vi "Configure TRIP.vi"(7 "All Channels (F)":bool, 8 "error in (no error)":errorcluster, 9 "Trip (0.00 s)":sgl format="%.2g", 10 "Channel (0)":u8, 11 "BoardHandle":T1) -> (0 "error out":errorcluster, 3 "BoardHandle out":T1)   [LabVIEW 2019, in "CAEN PSM.lvlib"]
doc: "This function allows to configure Ouput Trip time."
uses:
  CAEN PSM.lvlib
  Private/BoardHandle.ctl
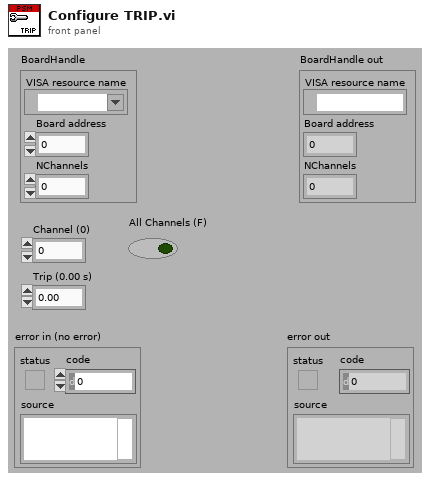
[diagram p1: front panel]
types:
  T1 = typedef "CAEN PSM.lvlib/BoardHandle.ctl" = cluster{"VISA resource name":refnum<visa-resource-name>, "Board address":u8, "NChannels":u8}
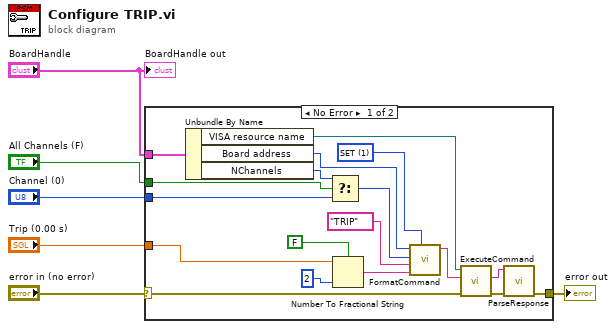
[diagram p0: block diagram]
diagram:
  n1 = case shown="No Error" "error in (no error)" {
    selector: "error in (no error)" -> [w12 w25]
    tunnel: "All Channels (F)" -> [w22 _]
    tunnel: "Channel (0)" -> [w20 _]
    tunnel: [w15 w25] -> w3
    tunnel: "BoardHandle" -> [w13 _]
    tunnel: "Trip (0.00 s)" -> [w7 _]
    frame No Error {
      w23 = u8 1 items=["MON", "SET"] ("CMD")
      n2 = Unbundle By Name(w13) -> ("VISA resource name"=w18:refnum<visa-resource-name>, "Board address"=w24:u8, "NChannels"=w21:u8)
      n3 = Select(t=w21, s=w22, f=w20) -> (s? t:f=w19:u8)
      n4 = Number To Fractional String(use system decimal point (T)=FALSE, number=w7, precision (6)=i16 2) -> (F-format string=w8:string)  [unwired: 1 in]
      n5 = call "FormatCommand.vi"("CMD (MON)"=w23, "VAL"=w8, "PAR"="TRIP", "CH"=w19, "BD (0)"=w24) -> ("cmd"=w17:string)  [unwired: 6 in]
      n6 = call "ExecuteCommand.vi"("error in (no error)"=w12, "Command"=w17, "VISA resource name"=w18) -> ("error out"=w16:errorcluster, "Response"=w14:string)  [unwired: 6 in, 1 out]
      n7 = call "ParseResponse.vi"("error in (no error)"=w16, "Response"=w14) -> ("error out"=w15:errorcluster)  [unwired: 6 in, 3 out]
    }
    frame Error {
    }
  }
  "error out" <- w3
  "BoardHandle out" <- "BoardHandle"
